vi "GetAlarmStatus.vi"(8 "error in":errorcluster, 10 "Channel Number":T1=1 items=["Channel 1"=1, "Channel 2"=2, "Channel 3"=3, "Channel 4"=4, "Channel 5"=5, "Channel 6"=6, "Channel 7"=7, "Channel 8"=8], 11 "VISA resource name":refnum<visa-resource-name>) -> (0 "error out":errorcluster, 1 "Alarm status":i32, 2 "Alarm status string":string, 3 "VISA resource name out":refnum<visa-resource-name>)   [LabVIEW 2023, in "Thermotron 8800.lvlib"]
doc: "ALRM\n\nCommand name: Alarm status\nCommand type: System status\nDescription: \nThe 8800 returns the current alarm status for the selected channel. The alarm status is a coded integer type as defined below:\n\nBit # Definition Bit # Definition\n0 Low deviation alarm\n1 High deviation alarm\n2 Not used\n3 Not used\n4 Low process alarm\n5 High process alarm\n6 Not used\n7 Not used\nSyntax: ALRMn?\nWhere n is any process variable channel (1 to 8).\nData type: Coded integer Example: ALRM2?\n8800 response: 1 (Channel 2 high deviation alarm)"
uses:
  Thermotron 8800.lvlib
  Private/AnalogInputChannelNumber.ctl
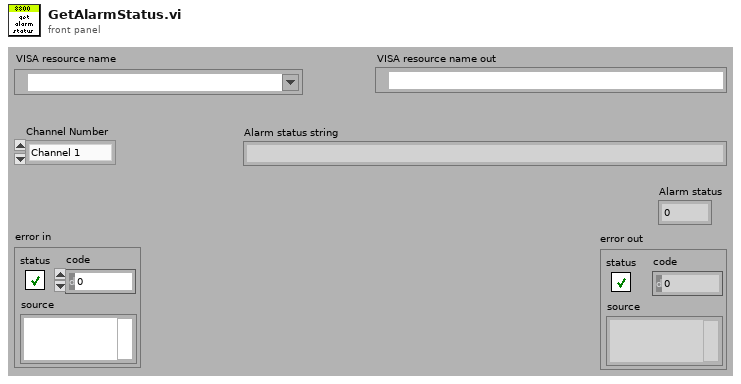
[diagram p1: front panel]
types:
  T1 = typedef "Thermotron 8800.lvlib/AnalogInputChannelNumber.ctl" = u16
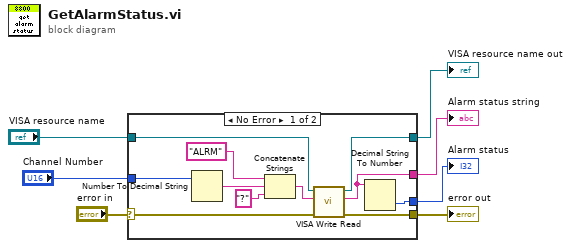
[diagram p0: block diagram]
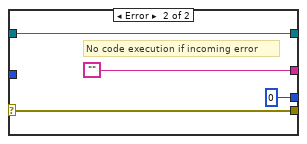
[diagram p2: hidden frame]
diagram:
  n1 = case shown="No Error" "error in" {
    selector: "error in" -> [w14 w22]
    tunnel: [w13 w22] -> w6
    tunnel: "Channel Number" -> [w12 _]
    tunnel: "VISA resource name" -> [w11 w19]
    tunnel: [w10 w19] -> w3
    tunnel: [w9 ""] -> w2
    tunnel: [w8 0] -> w1
    frame No Error {
      n2 = Number To Decimal String(number=w12) -> (decimal integer string=w18:string)  [unwired: 1 in]
      n3 = Concatenate Strings("ALRM" ("8800 Command"), w18, "?" ("8800 Command")) -> (w17:string)
      n4 = call "VISA Write Read.vi"("error in (no error)"=w14, "8800 Command"=w17, "VISA Refnum in"=w11) -> ("error out"=w13:errorcluster, "read buffer"=w9:string, "VISA Refnum out"=w10:refnum<visa-resource-name>)  [unwired: 6 in]
      n5 = Decimal String To Number(string=w9) -> (number=w8:i32)  [unwired: 2 in, 1 out]
    }
    frame Error {
      # "No code execution if incoming error"
    }
  }
  "error out" <- w6
  "VISA resource name out" <- w3
  "Alarm status string" <- w2
  "Alarm status" <- w1
